vi "DWF MSO Read.vi"(0 "Instrument Handle In":u32, 11 "Error In":errorcluster caption="Error In (no error)") -> (4 "Instrument Handle Out":u32, 6 "Analog Waveforms":waveform(dbl)[](array[waveform]), 8 "Digital Waveform":digitalwaveform(waveform)={"t0"=timestamp(0 s since 1904-01-01), "dt"=0.0, "Y"={"transitions"=[], "data"=[]}, "error"={"status"=FALSE, "code"=37421928, "source"=""}}, 10 "Trigger Time Stamp":timestamp, 14 "Trigger Reason":i32(ring) items=["Normal", "Forced", "Auto"], 15 "Error Out":errorcluster)   [LabVIEW 2015, in "DigilentWF.lvlib"]
doc: "Transfers data from the instrument as long as the acquisition state is Acquisition Complete. If the state is either Running or Triggered, this VI will wait until the state transitions to Acquisition Complete. If the state is Stopped, this VI returns an error."
uses:
  <vilib>/DigilentWF/DigilentWF.lvlib
  <vilib>/Waveform/DWDTOps.llb/DWDT Binary U16 to Digital.vi
  dwf.dll
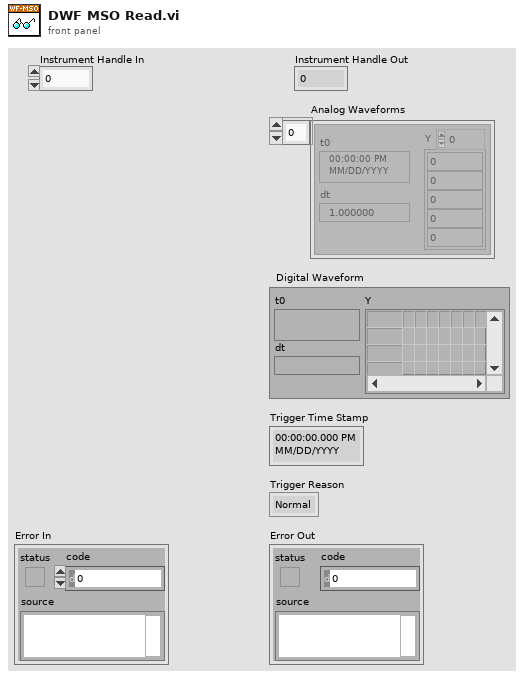
[diagram p1: front panel]
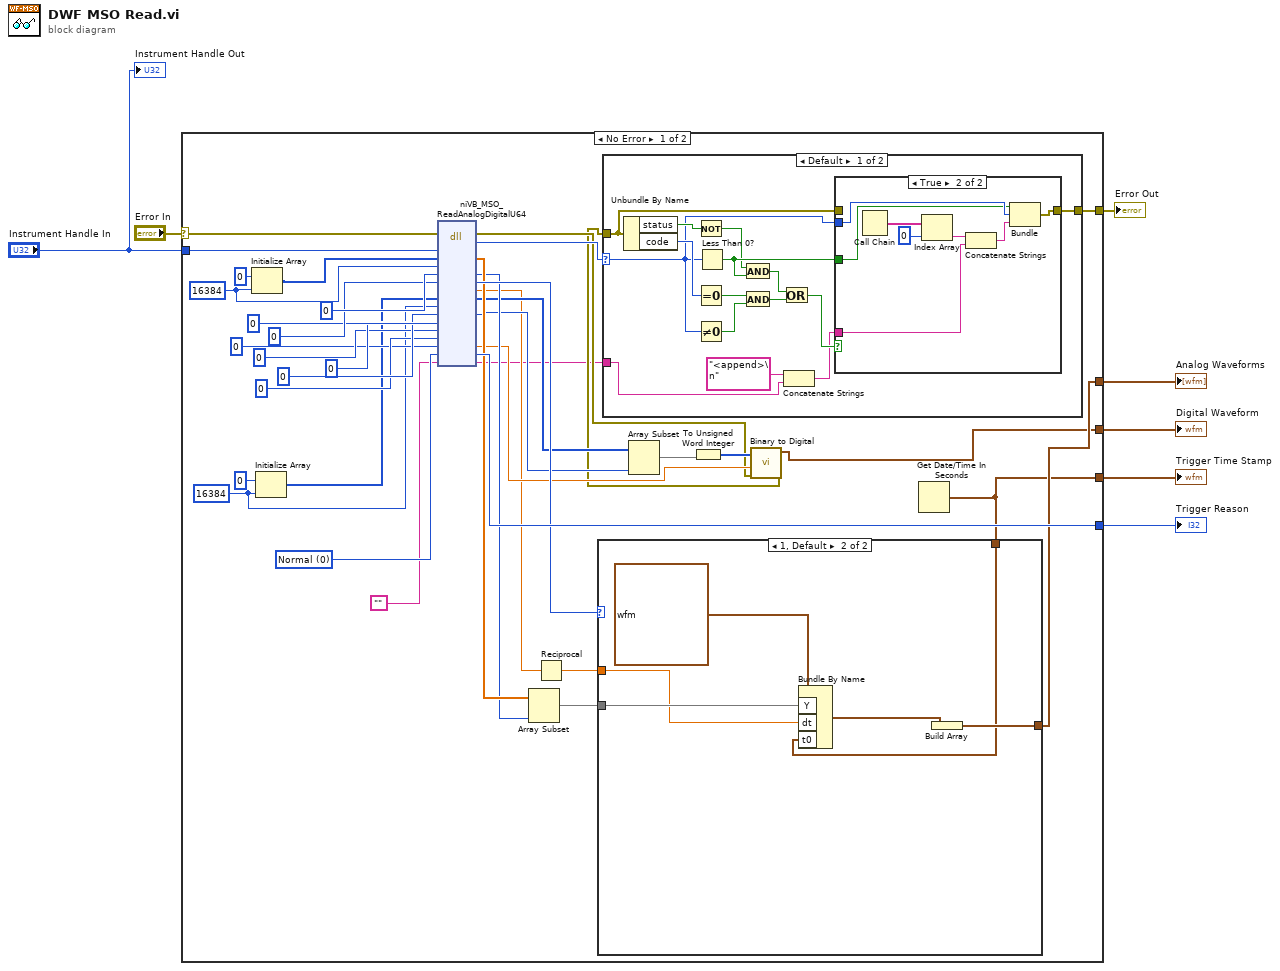
[diagram p0: block diagram]
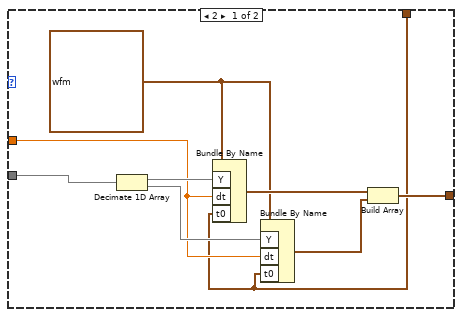
[diagram p2: hidden frame]
diagram:
  n1 = case "outter_case" shown="No Error" "Error In" {
    selector: "Error In" -> [w44 w86]
    tunnel: [w45 w86] -> w6
    tunnel: "Instrument Handle In" -> [w42 _]
    tunnel: [w28 _] -> w4
    tunnel: [w24 _] -> w3
    tunnel: [w12 _] -> w2
    tunnel: [w40 _] -> w1
    frame No Error {
      w19 = 16384 ("dimension size")
      w16 = 16384 ("dimension size")
      w41 = 0 items=["Normal", "Forced", "Auto"] ("Trigger Reason")
      n2 = Initialize Array(0, w16) -> (w30:i32[])
      n3 = Initialize Array(u64 0 ("element"), w19) -> (w22:u64[])
      n4 = dll-call lib="dwf.*" fn="niVB_MSO_ReadAnalogDigitalU64"(error in=w44, "instrumentHandle"=w42, "analogData"=w30, "analogDataSize"=w16, "analogDataSizeOut"=0, "analogDataStride"=0, "analogRate"=0 ("analogInitialTimestamp"), "digitalData"=w22, "digitalDataSize"=w19, "digitalDataSizeOut"=0, "digitalSampleTimestamps"=u32 0, "digitalSampleTimestampsSize"=0, "digitalSampleTimestampsSizeOut"=0, "digitalRate"=0 ("digitalInitialTimestamp"), "triggerReason"=w41, "szError"="") -> (error out=w14:errorcluster, "return type"=w43:i32, "analogData"=w27:dbl[], "analogDataSizeOut"=w26:i32, "analogDataStride"=w29:i32, "analogRate"=w11:dbl, "digitalData"=w21:u64[], "digitalDataSizeOut"=w20:i32, "digitalRate"=w15:dbl, "triggerReason"=w40:u32, "szError"=w8:string)  [unwired: 8 in, 1 out]
      n5 = Array Subset(array=w27, length=w26) -> (w25:dbl[])  [unwired: 1 in]
      n6 = Reciprocal(x=w11) -> (1/x=w10:dbl)
      n7 = Array Subset(array=w21, length=w20) -> (w17:u64[])  [unwired: 1 in]
      n8 = To Unsigned Word Integer(number=w17) -> (unsigned 16bit integer=w18:u16[])
      n9 = call-poly <vilib>:"Binary to Digital.vi"("error in (no error)"=w14, "sample rate"=w15, "binary array"=w18) -> ("error out"=w13:errorcluster, "digital waveform"=w24:digitalwaveform)  [unwired: 7 in]
      n10 = case "inner_case" shown="Default" w43 {
        selector: w43 -> [w65 _]
        tunnel: w13 -> [w66 w85]
        tunnel: [w62 w85] -> w45
        tunnel: w8 -> [w61 _]
        frame Default {
          n11 = Unbundle By Name(w66) -> ("status"=w70:bool, "code"=w74:i32)
          n12 = Not(x=w70) -> (.not. x?=w73:bool)
          n13 = Equal To 0?(x=w74) -> (x = 0?=w69:bool)
          n14 = Not Equal To 0?(x=w65) -> (x != 0?=w72:bool)
          n15 = Less Than 0?(x=w65) -> (x < 0?=w75:bool)
          n16 = And(x=w73, y=w75) -> (x .and. y?=w71:bool)
          n17 = And(x=w69, y=w72) -> (x .and. y?=w68:bool)
          n18 = Or(x=w71, y=w68) -> (x .or. y?=w67:bool)
          n19 = Concatenate Strings("<append>\n" ("string"), w61) -> (w64:string)
          n20 = case shown="True" w67 {
            tunnel: [w76 w83] -> w62
            tunnel: w65 -> [_ w82]
            tunnel: w75 -> [_ w81]
            tunnel: w66 -> [w76 _]
            tunnel: w64 -> [_ w77]
            frame False {
            }
            frame True {
              n21 = Call Chain() -> (call chain=w80:string[])
              n22 = Index Array(array=w80, index=0) -> (element=w79:string)
              n23 = Concatenate Strings(w79, w77) -> (w84:string)
              n24 = Bundle(w81, "return type"=w82, w84) -> (w83:cluster{bool, "return type":i32, string})  [unwired: 1 out]
            }
          }
        }
        frame 0 {
        }
      }
      n25 = Get Date/Time In Seconds() -> (seconds since 1Jan1904=w12:timestamp)
      n26 = case shown="1, Default" w29 {
        tunnel: w25 -> [w48 w57]
        tunnel: [w53 w59] -> w28
        tunnel: w10 -> [w47 w56]
        tunnel: w12 -> [w46 w55]
        frame 2 {
          w51 = waveform(dbl) {"t0"=timestamp(0 s since 1904-01-01), "dt"=1.0, "Y"=[]} ("Waveform")
          n27 = Decimate 1D Array(w48) -> (w50:dbl[], w49:dbl[])
          n28 = Bundle By Name(cluster=w51, "Y"=w50, "dt"=w47, "t0"=w46) -> (w54:waveform(dbl))
          n29 = Bundle By Name(cluster=w51, "Y"=w49, "dt"=w47, "t0"=w46) -> (w52:waveform(dbl))
          n30 = Build Array(w54, w52) -> (w53:waveform(dbl)[])
        }
        frame 1, Default {
          n31 = Bundle By Name(cluster=waveform(dbl) {"t0"=timestamp(0 s since 1904-01-01), "dt"=1.0, "Y"=[]} ("Waveform"), "Y"=w57, "dt"=w56, "t0"=w55) -> (w60:waveform(dbl))
          n32 = Build Array(w60) -> (w59:waveform(dbl)[])
        }
      }
    }
    frame Error {
    }
  }
  "Error Out" <- w6
  "Analog Waveforms" <- w4
  "Digital Waveform" <- w3
  "Trigger Time Stamp" <- w2
  "Trigger Reason" <- w1
  "Instrument Handle Out" <- "Instrument Handle In"
